vi "Start Server.vi"(8 "error in":errorcluster, 11 "port (54444)":u16=54444) -> (0 "error out":errorcluster)   [LabVIEW 2010, in "NI_CCC.lvlib"]
doc: "Asynchronously runs an instance of the CCC server process. One instance of the CCC server can be run for each unique port number."
uses:
  NI_CCC.lvlib
  FG Server Instances Action.ctl
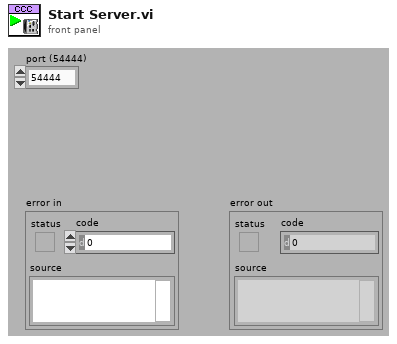
[diagram p1: front panel]
types:
  T1 = typedef "NI_CCC.lvlib/FG Server Instances Action.ctl" = enum16{"Find Instance", "Find All", "Register Instance", "Unregister Instance", "Unregister All"}
  T2 = enum32{"Bad", "Idle", "Run top level", "Running"}
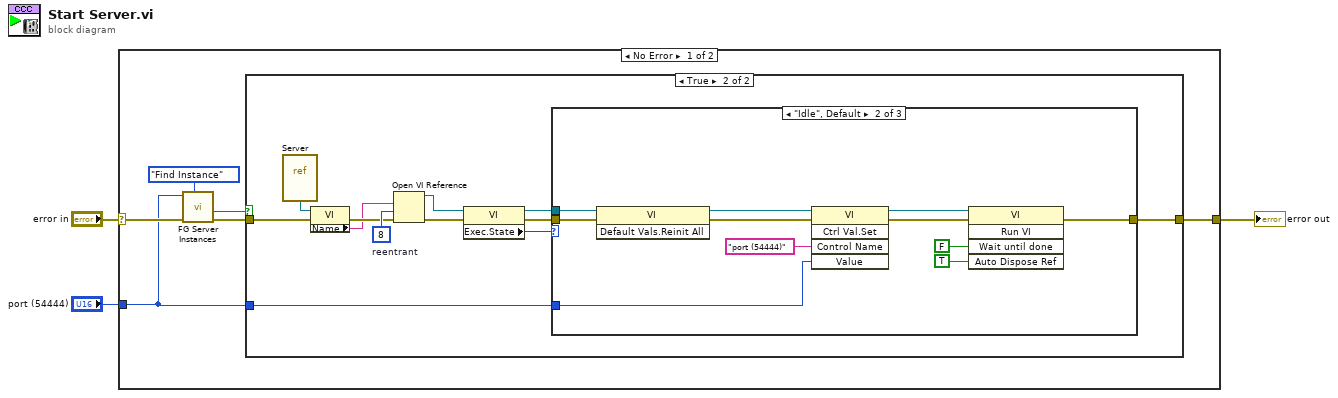
[diagram p0: block diagram]
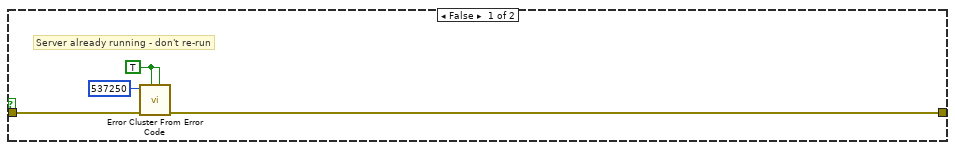
[diagram p2: hidden frame]
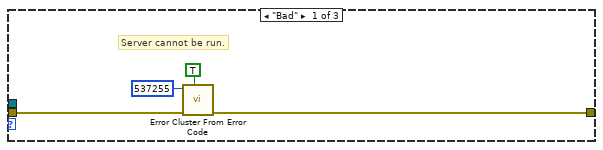
[diagram p3: hidden frame]
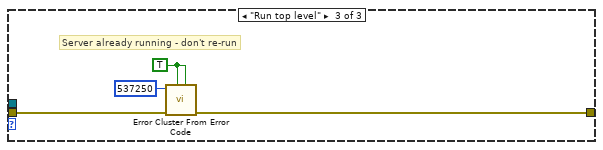
[diagram p4: hidden frame]
diagram:
  n1 = case shown="No Error" "error in" {
    selector: "error in" -> [w8 w45]
    tunnel: [w9 w45] -> w2
    tunnel: "port (54444)" -> [w6 _]
    frame No Error {
      n2 = call "FG Server Instances.vi"("action"=FG_Server_Instances_Action."Find Instance", "error in"=w8, "port"=w6) -> ("error out"=w5:errorcluster, "failed?"=w4:bool)  [unwired: 5 in, 2 out]
      n3 = case shown="True" w4 {
        tunnel: [w11 w25] -> w9
        tunnel: w6 -> [_ w22]
        tunnel: w5 -> [w12 w21]
        frame False {
          w10 = TRUE ("is warning? (False)")
          # "Server already running - don't re-run"
          n4 = call <vilib>:"Error Cluster From Error Code.vi"("is warning? (False)"=w10, "show call chain? (False)"=w10, "error in (no error)"=w12, "error code (0)"=537250) -> ("error out"=w11:errorcluster)  [unwired: 5 out]
        }
        frame True {
          w18 = 8  # reentrant
          n5 = vi-ref "Server.vi"() -> (w17:refnum<vi>)
          n6 = property class="VI"(reference=w17, error in=w21) -> (error out=w16:errorcluster, "Name"=w15:string)  [unwired: 1 out]
          n7 = Open VI Reference(vi path=w15, options=w18, error in (no error)=w16) -> (vi reference=w19:refnum<vi>, error out=w20:errorcluster)  [unwired: 3 in]
          n8 = property class="VI"(reference=w19, error in=w20) -> (reference out=w24:refnum<vi>, error out=w23:errorcluster, "Exec.State"=w14:T2)
          n9 = case shown="\"Idle\", Default" w14 {
            tunnel: [w27 w40 w42] -> w25
            tunnel: w24 -> [_ w39 _]
            tunnel: w23 -> [w28 w38 w43]
            tunnel: w22 -> [_ w32 _]
            frame "Bad" {
              # "Server cannot be run."
              n10 = call <vilib>:"Error Cluster From Error Code.vi"("show call chain? (False)"=TRUE, "error in (no error)"=w28, "error code (0)"=537255) -> ("error out"=w27:errorcluster)  [unwired: 6 out]
            }
            frame "Idle", Default {
              n11 = invoke class="VI" method="Default Vals.Reinit All"(reference=w39, error in=w38) -> (reference out=w36:refnum<vi>, error out=w35:errorcluster)  [unwired: 1 in, 1 out]
              n12 = invoke class="VI" method="Ctrl Val.Set"(reference=w36, error in=w35, "Control Name"="port (54444)", "Value"=w32) -> (reference out=w34:refnum<vi>, error out=w33:errorcluster)  [unwired: 1 in, 3 out]
              n13 = invoke class="VI" method="Run VI"(reference=w34, error in=w33, "Wait until done"=FALSE ("Wait Until Done"), "Auto Dispose Ref"=TRUE ("Auto Dispose Reference")) -> (error out=w40:errorcluster)  [unwired: 1 in, 4 out]
            }
            frame "Run top level" {
              w41 = TRUE ("is warning? (False)")
              # "Server already running - don't re-run"
              n14 = call <vilib>:"Error Cluster From Error Code.vi"("is warning? (False)"=w41, "show call chain? (False)"=w41, "error in (no error)"=w43, "error code (0)"=537250) -> ("error out"=w42:errorcluster)  [unwired: 5 out]
            }
          }
        }
      }
    }
    frame Error {
    }
  }
  "error out" <- w2
